vi "Untitled 2.vi"() -> ()   [LabVIEW 2013]
uses:
  <vilib>/sound2/lvsound2.llb/Sampling Mode.ctl
  <vilib>/sound2/lvsound2.llb/Sound Data Format.ctl
  <vilib>/sound2/lvsound2.llb/Sound Output Set Volume (Single).vi
  <vilib>/sound2/lvsound2.llb/Sound Output Write (DBL Single).vi
panel:
  in  "Amplitude":dbl=1.0
  in  "Enable 2":bool caption="Enable"
  in  "Enable":bool
  in  "Device ID":u32
  in  "Stop":bool
  in  "Frequency":dbl=500.0
  out "Generated Sound":waveform(dbl)(graph)
  in  "Volume":dbl(slide)=50.0 scale=0.0..100.0
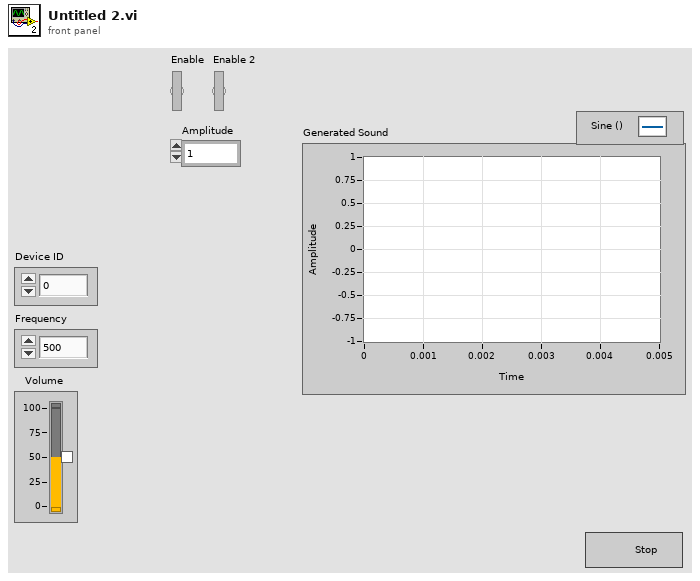
[diagram p1: front panel]
types:
  T1 = typedef "Sound Data Format.ctl" = cluster{"sample rate (S/s)":dbl, "number of channels":i32, "bits per sample":i32}
  T2 = typedef "Sampling Mode.ctl" = i32
  T3 = typedef "Sound Output Task ID.ctl" = u32
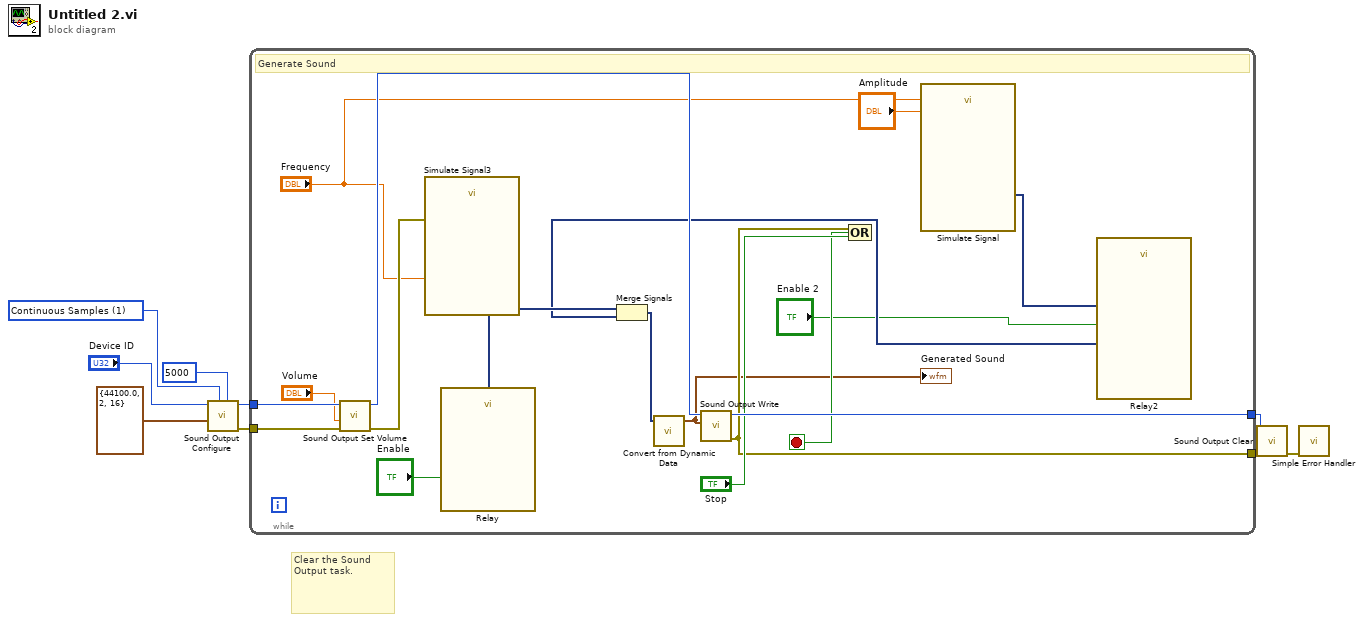
[diagram p0: block diagram]
diagram:
  w4 = T2 1 items=["Finite Samples", "Continuous Samples"] ("sample mode")
  # "Clear the Sound Output task."
  n1 = call <vilib>:"Sound Output Configure.vi"("number of samples/ch"=5000 ("Number of Samples/ch"), "sample mode"=w4, "sound format"=T1 {"sample rate (S/s)"=44100.0, "number of channels"=2, "bits per sample"=16} ("Sound Format"), "device ID"="Device ID") -> ("error out"=w9:errorcluster, "task ID"=w8:T3)  [unwired: 6 in]
  n2 = while {
    tunnel: w8 -> [w23]
    tunnel: [w28] -> w6
    tunnel: w9 -> [w25]
    tunnel: [w21] -> w7
    stop <- w26 stop-if-true
    # "Generate Sound"
    n3 = call-poly <vilib>:"Sound Output Set Volume.vi"("error in (no error)"=w25, "volume"="Volume", "task ID"=w23) -> ("error out"=w19:errorcluster, "task ID out"=w24:T3)  [unwired: 7 in]
    n4 = call "Simulate Signal3"("Frequency"="Frequency", "error in (no error)"=w19) -> ("Sine"=w18:dynamicdata)  [unwired: 12 in, 1 out]
    n5 = call "Relay"("Enable"="Enable", "Signals"=w18) -> ("Result"=w14:dynamicdata)  [unwired: 8 in, 1 out]
    n6 = call "Simulate Signal"("Frequency"="Frequency", "Amplitude"="Amplitude") -> ("Square"=w15:dynamicdata)  [unwired: 12 in, 1 out]
    n7 = call "Relay2"("Enable"="Enable 2", "Signals"=w15) -> ("Result"=w12:dynamicdata)  [unwired: 8 in, 1 out]
    n8 = Merge Signals(w14, w12) -> (w16:dynamicdata)
    n9 = call "Convert from Dynamic Data"("Dynamic Data Type"=w16) -> ("Waveform"=w20:waveform(dbl))  [unwired: 3 in]
    "Generated Sound" <- w20
    n10 = call-poly <vilib>:"Sound Output Write.vi"("data"=w20, "task ID"=w24) -> ("error out"=w21:errorcluster, "task ID out"=w28:T3)  [unwired: 8 in]
    n11 = Compound Arithmetic op=OR(w21, "Stop") -> (w26:bool)
  }
  n12 = call <vilib>:"Sound Output Clear.vi"("error in (no error)"=w7, "task ID"=w6) -> ("error out"=w2:errorcluster)  [unwired: 9 in]
  n13 = call <vilib>:"Simple Error Handler.vi"("error in (no error)"=w2) -> ()  [unwired: 4 in, 5 out]
